vi "Reset Waveform DVRs.vi"(8 "error in (no error)":errorcluster, 10 "Number of Waveforms":i32=-2, 11 "DVR Circular Buffer in":refnum<data-value>[](array[refnum])) -> (0 "error out":errorcluster, 3 "DVR Circular Buffer out":refnum<data-value>[](array[refnum]))   [LabVIEW 2021, in "CIF_NIChn_FIFO_DAQ_DVR.lvclass"]
uses:
  CIF_NIChn_FIFO_DAQ_DVR.lvclass
  ChannelCommon/typedef/Datatype Waveform.ctl
  ChannelCommon/ChannelCommon.lvlib
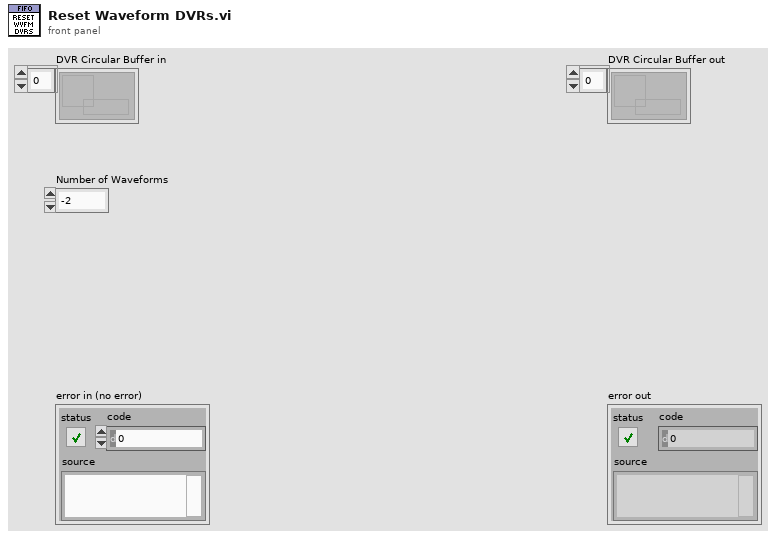
[diagram p1: front panel]
types:
  T1 = typedef "ChannelCommon.lvlib/Datatype Waveform.ctl" = cluster{"measurement":dbl[], "dT":dbl, "Timestamp":i64, "Read Lock":bool}
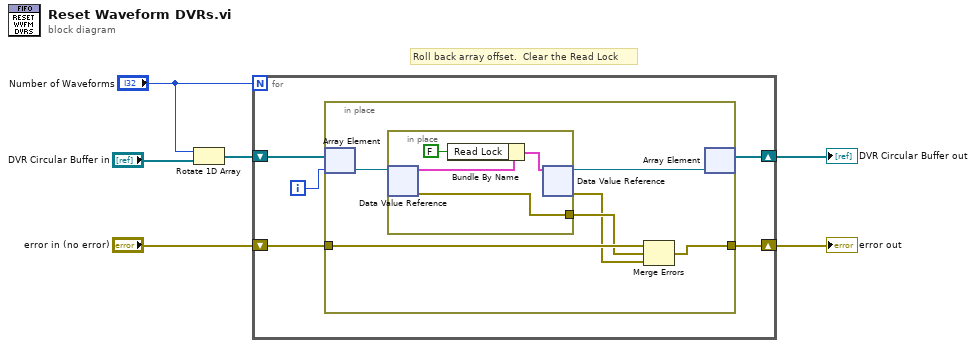
[diagram p0: block diagram]
diagram:
  # "Roll back array offset.  Clear the Read Lock"
  n1 = Rotate 1D Array(1:"DVR Circular Buffer in", 2:"Number of Waveforms") -> (0:w2:refnum<data-value>[])
  n2 = for {
    N: "Number of Waveforms" -> [_]
    shift-right: [w10] -> w4
    shift-left: "error in (no error)" -> [w11]
    shift-right: [w8] -> w1
    shift-left: w2 -> [w9]
    i -> [w7]
    n3 = in-place {
      in-place-border: w11 -> [w17]
      in-place-border: [w16] -> w10
      n4 = in-place-array #1(w9, w7) -> (w15:refnum<data-value>)
      n5 = in-place {
        in-place-border: [w21] -> w13
        n6 = in-place-dvr #2(w15) -> (w20:T1, w21:errorcluster)
        n7 = Bundle By Name(cluster=w20, "Read Lock"=FALSE) -> (w19:T1)
        n8 = in-place-dvr #2(w19) -> (w14:refnum<data-value>, w12:errorcluster)
      }
      n9 = Merge Errors(w17, w13, w12) -> (w16:errorcluster)
      n10 = in-place-array #1(w14) -> (w8:refnum<data-value>[])  [unwired: 1 out]
    }
  }
  "error out" <- w4
  "DVR Circular Buffer out" <- w1
